vi "Generate frequencies map.vi"() -> ()   [LabVIEW 2019]
panel:
  out "Map":map{i16, dbl}(c390)
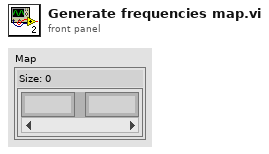
[diagram p1: front panel]
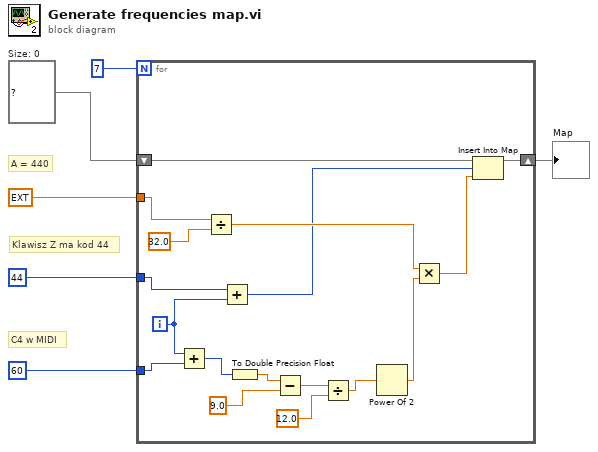
[diagram p0: block diagram]
diagram:
  w5 = map{i16, dbl} {}  # Size: 0
  # "Klawisz Z ma kod 44"
  # "C4 w MIDI"
  # "A = 440"
  n1 = for {
    N: 7 -> [_]
    shift-right: [w22] -> w1
    shift-left: w5 -> [w23]
    tunnel: 44 ("x") -> [w9]
    tunnel: 60 -> [w13]
    tunnel: ext 440.0 -> [w16]
    i -> [w8]
    n2 = Add(x=w8, y=w13) -> (x+y=w14:i32)
    n3 = Divide(x=w16, y=32.0) -> (x/y=w11:ext)
    n4 = Add(x=w9, y=w8) -> (x+y=w7:i32)
    n5 = To Double Precision Float(number=w14) -> (double precision float=w18:dbl)
    n6 = Subtract(x=w18, y=9.0) -> (x-y=w20:dbl)
    n7 = Divide(x=w20, y=12.0) -> (x/y=w17:dbl)
    n8 = Power Of 2(x=w17) -> (2^x=w12:dbl)
    n9 = Multiply(x=w11, y=w12) -> (x*y=w10:ext)
    n10 = Insert Into Map(map in=w23, key=w7, value=w10) -> (map out=w22:map{i16, dbl})  [unwired: 2 out]
  }
  "Map" <- w1
